vi "CheckDevice.vi"(6 "timeout (10000)":i32=10000, 8 "CheckVersion":bool, 9 "DevicesNames":string[](array[string]), 11 "DeviceList":T1[](array[typedef])) -> (0 "UpdatedDevices":T1[](array[typedef]), 1 "DevicesToUpdateNames":string[](array[string]), 2 "NotUpdatedDevicesNames":string[](array[string]), 3 "OnlineDevices":T1[](array[typedef]), 4 "UpdatedDevicesName":string[](array[string]), 5 "DevicesToUpdate":T1[](array[typedef]))   [LabVIEW 2016]
uses:
  <vilib>/addons/InsightCM/MessageBus/MessageLibrary/SysCfgDeployer/controls/SysCfgDeployPackageRequestBody.ctl
panel:
  out "millisecond timer value":u32
  out "IpAddress":string
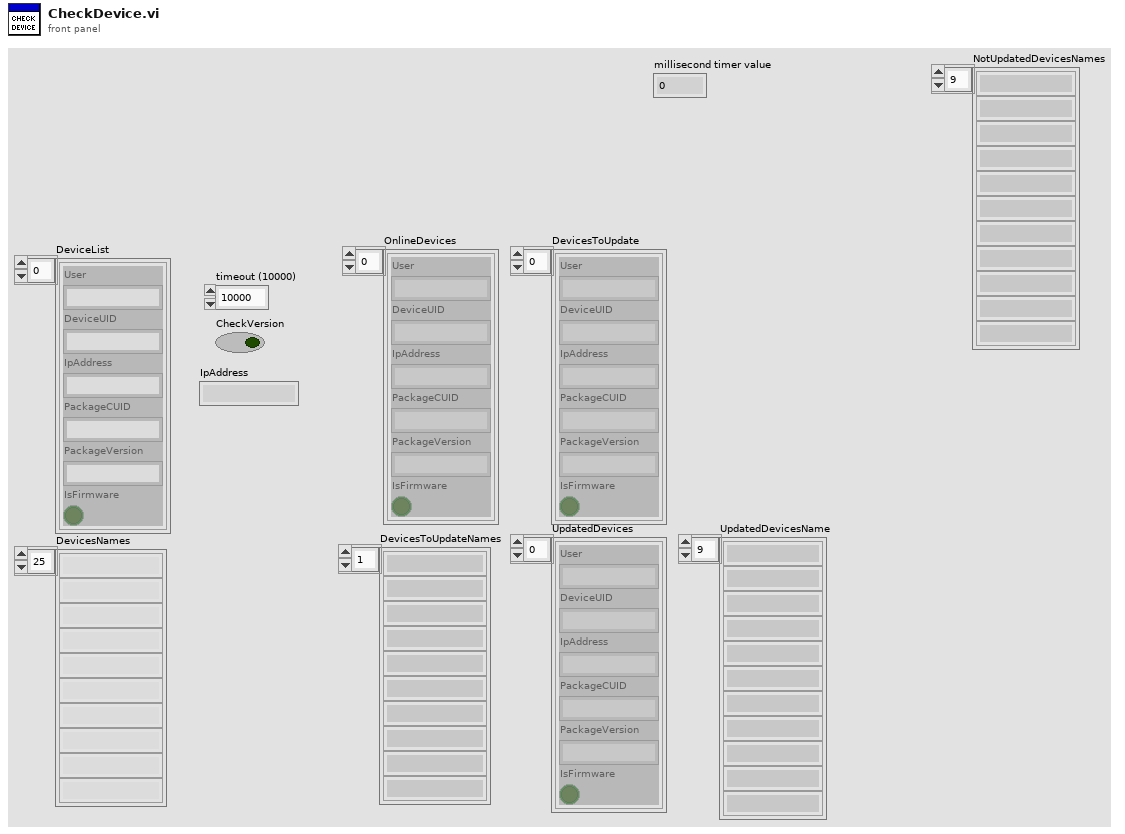
[diagram p1: front panel]
types:
  T1 = typedef "SysCfgDeployPackageRequestBody.ctl" = cluster{"User":string, "DeviceUID":string, "IpAddress":string, "PackageCUID":string, "PackageVersion":string, "IsFirmware":bool}
  T2 = cluster{"Title":string, "Description":string, "ID":string, "Version":string}
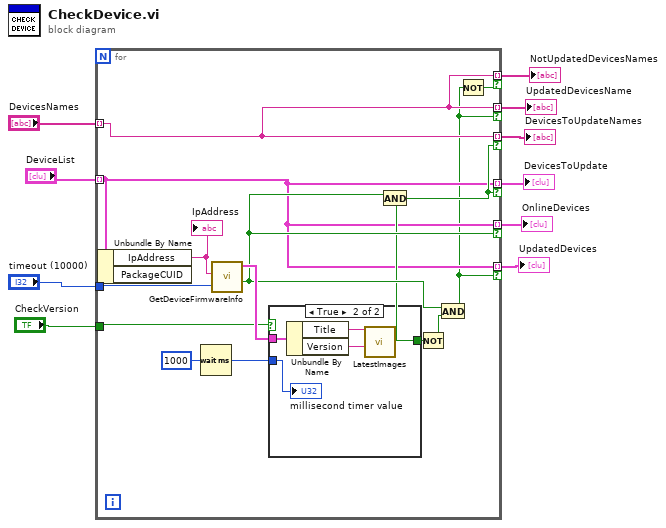
[diagram p0: block diagram]
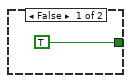
[diagram p2: hidden frame]
diagram:
  n1 = for {
    tunnel: "DeviceList" -> [w16] mode=indexing
    tunnel: [w15] -> w2 mode=indexing if=w13
    tunnel: [w16] -> w9 mode=indexing if=w18
    tunnel: [w16] -> w8 mode=indexing if=w22
    tunnel: "DevicesNames" -> [w15] mode=indexing
    tunnel: [w15] -> w6 mode=indexing if=w22
    tunnel: "timeout (10000)" -> [w21]
    tunnel: "CheckVersion" -> [w20]
    tunnel: [w16] -> w3 mode=indexing if=w13
    tunnel: [w15] -> w1 mode=indexing if=w14
    n2 = Unbundle By Name(w16) -> ("IpAddress"=w24:string)  [unwired: 1 out]
    "IpAddress" <- w24
    n3 = Wait (ms)(milliseconds to wait=u32 1000) -> (millisecond timer value=w11:u32)
    n4 = call "GetDeviceFirmwareInfo.vi"("timeout (10000)"=w21, "IP"=w24) -> ("ConnectedToWebService"=w18:bool, "AppVersion"=w23:T2)  [unwired: 8 in]
    n5 = case shown="True" w20 {
      tunnel: w23 -> [_ w30]
      tunnel: [TRUE ("y") w27] -> w17
      tunnel: w11 -> [_ w26]
      frame False {
      }
      frame True {
        n6 = Unbundle By Name(w30) -> ("Title"=w29:string, "Version"=w28:string)
        n7 = call "LatestImages.vi"("VersionInput"=w28, "ImageInput"=w29) -> ("Update"=w27:bool)  [unwired: 9 in]
        "millisecond timer value" <- w26
      }
    }
    n8 = And(x=w18, y=w17) -> (x .and. y?=w22:bool)
    n9 = Not(x=w17) -> (.not. x?=w19:bool)
    n10 = And(x=w18, y=w19) -> (x .and. y?=w13:bool)
    n11 = Not(x=w13) -> (.not. x?=w14:bool)
  }
  "OnlineDevices" <- w9
  "DevicesToUpdate" <- w8
  "DevicesToUpdateNames" <- w6
  "UpdatedDevices" <- w3
  "UpdatedDevicesName" <- w2
  "NotUpdatedDevicesNames" <- w1
